vi "Same Buffer.vi"(8 "error in (no error)":errorcluster, 10 "Buffer 2":refnum<class "Buffer.lvclass">, 11 "Buffer 1":refnum<class "Buffer.lvclass">) -> (0 "error out":errorcluster, 2 "same buffer?":bool)   [LabVIEW 2021, in "DSF Core.lvlib" / "Buffer.lvclass"]
uses:
  Buffer.lvclass
  C:/Program Files/National Instruments/LabVIEW 2021/vi.lib/NI/Memory Manager/Classes/Pointer/Pointer.lvclass
  <vilib>/NI/Memory Manager/Classes/Pointer/Pointer.lvclass/Pointer.ctl
  <vilib>/NI/Memory Manager/Classes/Pointer/Get Size.vi
  <vilib>/NI/Memory Manager/Classes/Pointer/Get Address.vi
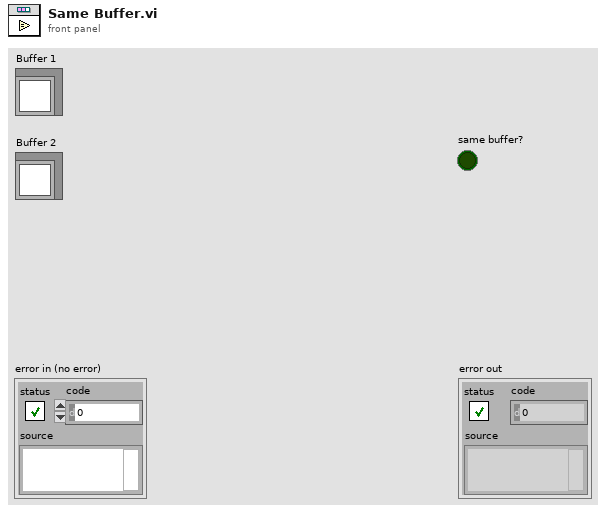
[diagram p1: front panel]
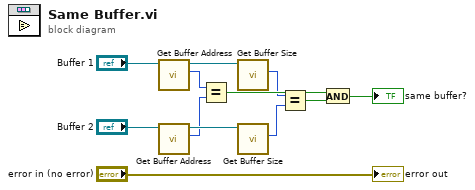
[diagram p0: block diagram]
diagram:
  n1 = call "Get Buffer Address.vi"("Buffer in"="Buffer 1") -> ("buffer address"=w7:u64, "Buffer out"=w11:refnum<class "Buffer.lvclass">)  [unwired: 9 in]
  n2 = call "Get Buffer Address.vi"("Buffer in"="Buffer 2") -> ("buffer address"=w6:u64, "Buffer out"=w9:refnum<class "Buffer.lvclass">)  [unwired: 9 in]
  n3 = Equal?(x=w7, y=w6) -> (x = y?=w4:bool)
  n4 = call "Get Buffer Size.vi"("Buffer in"=w11) -> ("buffer size"=w3:u64)  [unwired: 9 in, 1 out]
  n5 = call "Get Buffer Size.vi"("Buffer in"=w9) -> ("buffer size"=w2:u64)  [unwired: 9 in, 1 out]
  n6 = Equal?(x=w3, y=w2) -> (x = y?=w5:bool)
  n7 = And(x=w4, y=w5) -> (x .and. y?=→"same buffer?":bool)
  "error out" <- "error in (no error)"
